vi "UTILITY Type Conv Seconds Time String.vi"(8 "Time String In":string, 11 "Seconds In":dbl format="%<%H:%M:%S>t") -> (0 "Seconds Out":dbl, 3 "Time String Out":string)   [LabVIEW 2016]
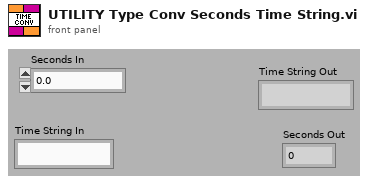
[diagram p1: front panel]
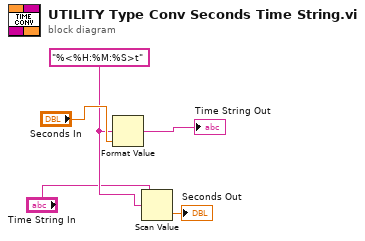
[diagram p0: block diagram]
diagram:
  w2 = "%<%H:%M:%S>t" ("string (\"\")")
  n1 = Format Value(format string=w2, value (0)="Seconds In") -> (output string=→"Time String Out":string)  [unwired: 1 in]
  n2 = Scan Value(string="Time String In", format string=w2) -> (value=→"Seconds Out":dbl)  [unwired: 1 in, 1 out]
